vi "SequenceIndexWrite.vi"(8 "error in (no error)":errorcluster, 9 "OriginalName":string, 10 "SequenceIndex":refnum<class "SequenceIndex.lvclass">, 11 "VariableManager in":refnum<class "VariableManager.lvclass">) -> (0 "error out":errorcluster, 3 "VariableManager out":refnum<class "VariableManager.lvclass">)   [LabVIEW 2013, in "VariableManager.lvclass"]
doc: "Add the given sequence index definition to database.\nTo overwrite existing sequence index definition, provide the OriginalName.\n\nAn error is thrown if the given SequenceIndex is malformed, failing the test in SequenceIndexCheck.vi\n\nSuppose that a sequence index has a name <B>idx</B>. Three names are reserved for uses in sequence function\n<B>idx</B>: Integer value that runs from 0 to (idx.Steps-1)\n<B>idx_f</B>: Double value that runs [0,1] (gives 0, if the idx.Steps is 1)\n<B>idx_max</B>: An integer equals to idx.Steps"
uses:
  VariableManager.lvclass
  SequenceIndex/SequenceIndex.lvclass
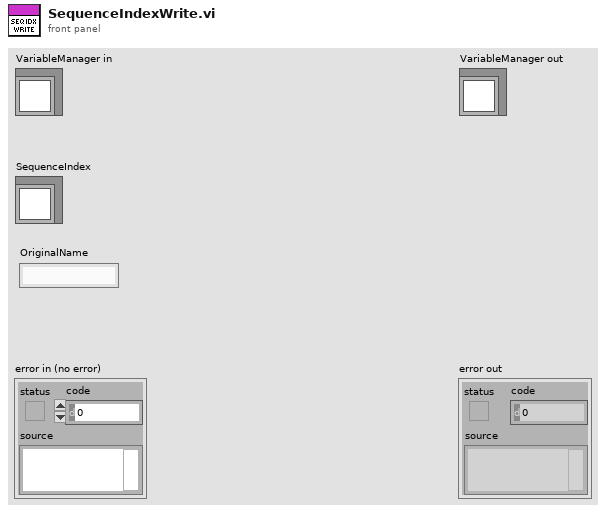
[diagram p1: front panel]
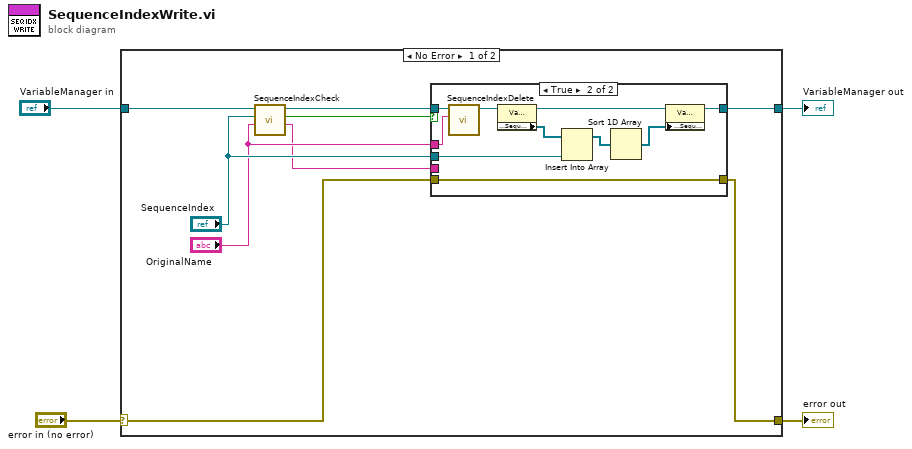
[diagram p0: block diagram]
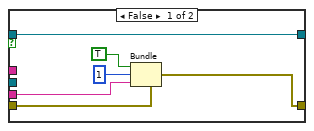
[diagram p2: hidden frame]
diagram:
  n1 = case shown="No Error" "error in (no error)" {
    selector: "error in (no error)" -> [w6 w31]
    tunnel: [w5 w31] -> w3
    tunnel: [w13 w30] -> w1
    tunnel: "VariableManager in" -> [w12 w30]
    frame No Error {
      n2 = call-dynamic "SequenceIndexCheck.vi"("OriginalName"="OriginalName", "SequenceIndex"="SequenceIndex", "VariableManager in"=w12) -> ("RejectMessage"=w7:string, "Pass"=w10:bool, "VariableManager out"=w11:refnum<class "VariableManager.lvclass">)  [unwired: 5 in, 1 out]
      n3 = case shown="True" w10 {
        tunnel: [w19 w25] -> w13
        tunnel: w11 -> [w19 w24]
        tunnel: "SequenceIndex" -> [_ w22]
        tunnel: "OriginalName" -> [_ w21]
        tunnel: w6 -> [w16 w20]
        tunnel: w7 -> [w15 _]
        tunnel: [w14 w20] -> w5
        frame False {
          n4 = Bundle(cluster=w16, "status"=TRUE, "code"=1, "source"=w15) -> (w14:errorcluster)
        }
        frame True {
          n5 = call-dynamic "SequenceIndexDelete.vi"("SequenceIndexName"=w21, "VariableManager in"=w24) -> ("VariableManager out"=w23:refnum<class "VariableManager.lvclass">)  [unwired: 8 in, 1 out]
          n6 = property class="VariableManager.lvclass"(reference=w23) -> (reference out=w29:refnum<class "VariableManager.lvclass">, "Accessors:SequenceIndices"=w28:refnum<class "SequenceIndex.lvclass">[])  [unwired: 1 in, 1 out]
          n7 = Insert Into Array(array=w28, new element=w22) -> (w27:refnum<class "SequenceIndex.lvclass">[])  [unwired: 1 in]
          n8 = Sort 1D Array(array=w27) -> (sorted array=w26:refnum<class "SequenceIndex.lvclass">[])
          n9 = property class="VariableManager.lvclass"(reference=w29, "Accessors:SequenceIndices"=w26) -> (reference out=w25:refnum<class "VariableManager.lvclass">)  [unwired: 1 in, 1 out]
        }
      }
    }
    frame Error {
    }
  }
  "error out" <- w3
  "VariableManager out" <- w1
